vi "SubVI_Collect_User_History.vi"(8 "error in (no error)":errorcluster, 9 "Goal (Sessions)":dbl, 10 "Goal (Trials)":dbl, 11 "Goal (Minutes)":dbl) -> (0 "error out":errorcluster)   [LabVIEW 2020]
uses:
  Global 1.vi
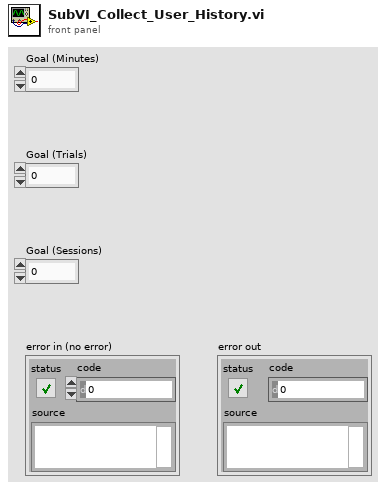
[diagram p1: front panel]
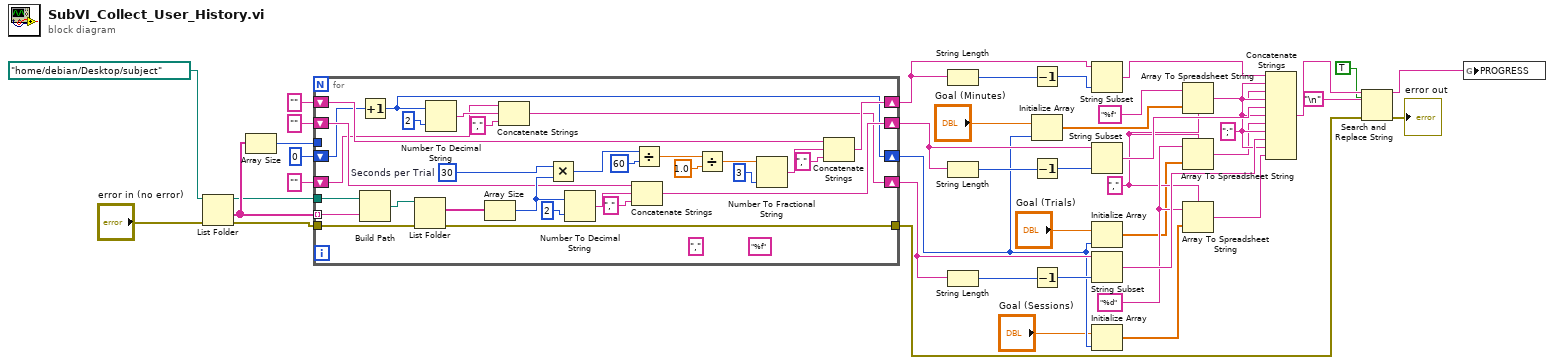
[diagram p0: block diagram]
diagram:
  w29 = "%d" ("format string")
  w25 = ";" ("string")
  w22 = "," ("delimiter (Tab)")
  n1 = List Folder(path=path "/home/debian/Desktop/subject" ("base path"), error in="error in (no error)") -> (path out=w3:path, folder names=w10:string[], error out=w4:errorcluster)  [unwired: 2 in, 1 out]
  n2 = Array Size(array=w10) -> (size(s)=w11:i32)
  n3 = for {
    tunnel: w10 -> [w72] mode=indexing
    tunnel: w3 -> [w71]
    tunnel: w4 -> [w69]
    shift-right: [w61] -> w35
    shift-left: "" -> [w62]
    tunnel: [w63] -> w8
    tunnel: w11 -> [_]
    shift-right: [w53] -> w36
    shift-left: "" -> [w54]
    shift-right: [w51] -> w33
    shift-left: 0 -> [w52]
    shift-right: [w47] -> w39
    shift-left: "" -> [w48]
    (unwired) "%f" ("format string")
    (unwired) "," ("delimiter (Tab)")
    w68 = 30  # Seconds per Trial
    n4 = Increment(x=w52) -> (x+1=w51:i32)
    n5 = Build Path(base path=w71, name or relative path=w72) -> (appended path=w70:path)
    n6 = List Folder(path=w70, error in=w69) -> (filenames=w46:string[], error out=w63:errorcluster)  [unwired: 2 in, 2 out]
    n7 = Number To Decimal String(number=w51, width (-)=i16 2) -> (decimal integer string=w49:string)
    n8 = Array Size(array=w46) -> (size(s)=w57:i32)
    n9 = Concatenate Strings(w48, w49, "," ("string")) -> (w47:string)
    n10 = Multiply(x=w68, y=w57) -> (x*y=w67:i32)
    n11 = Number To Decimal String(number=w57, width (-)=i16 2) -> (decimal integer string=w55:string)
    n12 = Concatenate Strings(w54, w55, "," ("string")) -> (w53:string)
    n13 = Divide(x=w67, y=60) -> (x/y=w65:dbl)
    n14 = Divide(x=w65, y=1.0) -> (x/y=w60:dbl)
    n15 = Number To Fractional String(number=w60, precision (6)=i16 3) -> (F-format string=w59:string)  [unwired: 2 in]
    n16 = Concatenate Strings(w62, w59, "," ("string")) -> (w61:string)
  }
  n17 = String Length(string=w35) -> (length=w34:i32)
  n18 = String Length(string=w36) -> (length=w37:i32)
  n19 = String Length(string=w39) -> (length=w38:i32)
  n20 = Decrement(x=w34) -> (x-1=w40:i32)
  n21 = Initialize Array("Goal (Minutes)", w33) -> (w19:dbl[])
  n22 = Decrement(x=w37) -> (x-1=w41:i32)
  n23 = Decrement(x=w38) -> (x-1=w42:i32)
  n24 = String Subset(string=w35, length (rest)=w40) -> (substring=w30:string)  [unwired: 1 in]
  n25 = String Subset(string=w36, length (rest)=w41) -> (substring=w31:string)  [unwired: 1 in]
  n26 = Initialize Array("Goal (Trials)", w33) -> (w20:dbl[])
  n27 = String Subset(string=w39, length (rest)=w42) -> (substring=w32:string)  [unwired: 1 in]
  n28 = Initialize Array("Goal (Sessions)", w33) -> (w21:dbl[])
  n29 = Array To Spreadsheet String(delimiter (Tab)=w22, array=w19, 3:"%f" ("format string")) -> (spreadsheet string=w23:string)
  n30 = Array To Spreadsheet String(delimiter (Tab)=w22, array=w20, 3:w29) -> (spreadsheet string=w24:string)
  n31 = Array To Spreadsheet String(delimiter (Tab)=w22, array=w21, 3:w29) -> (spreadsheet string=w26:string)
  n32 = Concatenate Strings(w30, w25, w23, w25, w31, w25, w24, w25, w32, w25, w26) -> (w27:string)
  n33 = Search and Replace String(replace all?=TRUE ("replace all? (F)"), input string=w27, search string="\n", error in=w8) -> (result string=w12:string, error out=→"error out":errorcluster)  [unwired: 4 in, 2 out]
  n34 = global write "Global 1.vi" "PROGRESS"(w12) -> ()
